vi "is_cluster.vi"(1 "ctrl ref":refnum<vi>) -> (0 "is page?":bool)   [LabVIEW 2015]
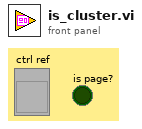
[diagram p1: front panel]
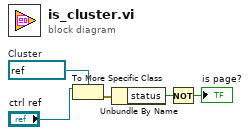
[diagram p0: block diagram]
diagram:
  w1 = refnum<vi> refnum  # Cluster
  n1 = To More Specific Class(target class=w1, reference="ctrl ref") -> (error out=w3:errorcluster)  [unwired: 1 in, 1 out]
  n2 = Unbundle By Name(w3) -> ("status"=w4:bool)
  n3 = Not(x=w4) -> (.not. x?=→"is page?":bool)
